vi "DiscArchiver.close file.vi"(0 "i ref in":refnum<vi>, 3 "ms timeout (10000)":i32=10000, 5 "error in (no error)":errorcluster) -> (14 "i ref out":refnum<vi>, 17 "timed out":bool, 19 "error out":errorcluster)   [LabVIEW 2014, in "DiscArchiver.lvlib"]
doc: "closes an open file."
uses:
  DiscArchiver.lvlib
  CSlibraries-extern/DimLVEvent/LVDimInterface/LVDimInterface.lvlib
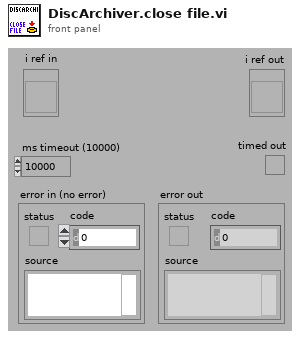
[diagram p1: front panel]
types:
  T1 = typedef "DiscArchiver.lvlib/DiscArchiver.i attribute.ctl" = cluster{"file prefix":string, "actual file":string, "nOfEvents":i32, "file":refnum<file>, "eventBuilder":string, "disc size alarm":bool, "dataDescription":string, "dataDescriptionURL":string, "eventDataURL":string, "headerID":dbl, "completeData":bool, "nOfEventsID":i32, "dataFileID":i32}
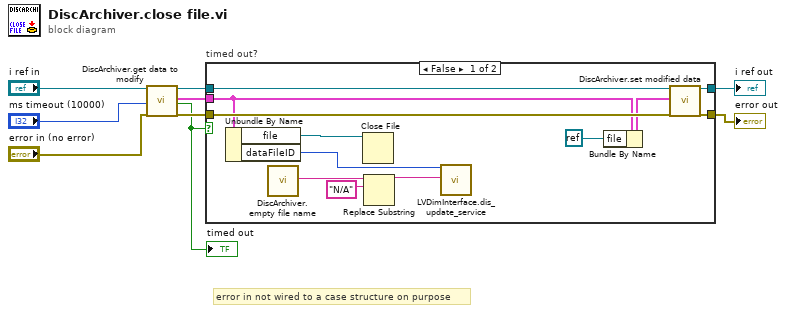
[diagram p0: block diagram]
diagram:
  # "error in not wired to a case structure on purpose"
  n1 = call "DiscArchiver.get data to modify.vi"("i ref in"="i ref in", "ms timeout (10000)"="ms timeout (10000)", "error in (no error)"="error in (no error)") -> ("i ref out"=w5:refnum<vi>, "i attribute"=w3:T1, "timed out"=w1:bool, "error out"=w4:errorcluster)  [unwired: 13 in]
  "timed out" <- w1
  n2 = case "timed out?" shown="False" w1 {
    tunnel: [w21 w22] -> w7
    tunnel: [w20 w23] -> w6
    tunnel: w5 -> [w19 w23]
    tunnel: w4 -> [w18 w22]
    tunnel: w3 -> [w16 _]
    frame False {
      n3 = Unbundle By Name(w16) -> ("file"=w15:refnum<file>, "dataFileID"=w13:i32)
      n4 = call "DiscArchiver.empty file name.vi"() -> ("emptyString"=w12:string)  [unwired: 19 in]
      n5 = Close File(refnum=w15) -> ()  [unwired: 1 in, 2 out]
      n6 = Replace Substring(4:"N/A" ("substring (\"\")"), 5:w12) -> (1:w10:string)  [unwired: 2 in, 1 out]
      n7 = call "LVDimInterface.dis_update_service.vi"("my_serviceID"=w13, "data"=w10) -> ()  [unwired: 15 in, 3 out]
      n8 = Bundle By Name(cluster=w16, "file"=refnum<k0> refnum) -> (w17:T1)
      n9 = call "DiscArchiver.set modified data.vi"("i ref in"=w19, "i attribute"=w17, "error in (no error)"=w18) -> ("i ref out"=w20:refnum<vi>, "error out"=w21:errorcluster)  [unwired: 15 in]
    }
    frame True {
    }
  }
  "error out" <- w7
  "i ref out" <- w6
